vi "Create Transceiver.vi"(5 "FIFO Debug Flags":refnum<class "Debug Flags FIFO.lvclass">, 7 "fifo depths (10)":u32=10, 8 "error in (no error)":errorcluster, 10 "error size (512 B)":T1=enum."512-byte", 11 "Transceiver Interface type":refnum<class "Transceiver Interface.lvclass">) -> (0 "error out":errorcluster, 3 "Transceiver Interface":refnum<class "Transceiver Interface.lvclass">)   [LabVIEW 2017, in "Data Sharing Framework Engine.lvlib" / "Transceiver Interface.lvclass"]
uses:
  Transceiver Interface.lvclass
  C:/github/data-sharing-framework/Source/Data Sharing Framework Core/Engine/Interfaces/Data Sharing Engine/Engine Interface.lvclass
  Engine Interface/Error Queue Sizes.ctl
  Debug/Debug Flags FIFO/Debug Flags FIFO.lvclass
  Engine Interface/Engine Interface.lvclass
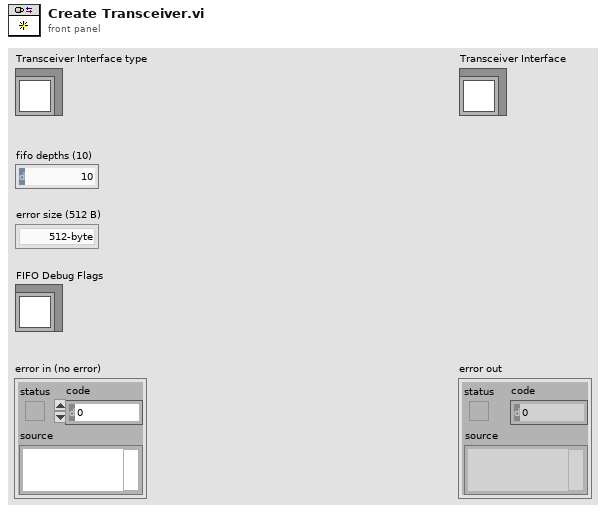
[diagram p1: front panel]
types:
  T1 = typedef "Data Sharing Framework Engine.lvlib/Engine Interface.lvclass/Error Queue Sizes.ctl" = enum16{"256-byte", "512-byte", "1024-byte"}
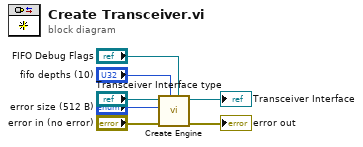
[diagram p0: block diagram]
diagram:
  n1 = call "Create Engine.vi"("FIFO Debug Flags"="FIFO Debug Flags", "fifo/queue depths (10)"="fifo depths (10)", "error in (no error)"="error in (no error)", "error size (512 B)"="error size (512 B)", "Interface type"="Transceiver Interface type") -> ("error out"=→"error out":errorcluster, "Interface"=→"Transceiver Interface":refnum<class "Transceiver Interface.lvclass">)  [unwired: 5 in]
